vi "Test Get Skip Result.vi"(8 "error in (no error)":errorcluster, 11 "Test Case In":refnum<class "Test Case V2 Test.lvclass">) -> (0 "error out":errorcluster, 3 "Test Case Out":refnum<class "Test Case V2 Test.lvclass">)   [LabVIEW 2020, in "Test Case V2 Test.lvclass"]
uses:
  Test Case V2 Test.lvclass
  C:/Program Files (x86)/National Instruments/LabVIEW 2020/vi.lib/Astemes/LUnit/Test Case.lvclass
  LUnit Test Case V2 Test Double/LUnit Test Case V2 Test Double.lvclass
  C:/Git/astemes-lunit/source/Rewrite Project/LUnit Test Case/LUnit Test Case V2.lvclass
  Framework/Result Types/Assertion Result/Public/TypeDefs/Status.ctl
  <vilib>/Astemes/LUnit/Test Case.lvclass/Test Case.ctl
  d765b41f-6b96-4a08-8de0-d57f3ce312ff.vi
  <vilib>/Astemes/LUnit/Palette/Pass.vi
  <vilib>/Astemes/LUnit/Palette/Fail.vi
  <vilib>/Astemes/LUnit/Compare Variants.vi
  <vilib>/Astemes/LUnit/Describe Comparison.vi
  <vilib>/Astemes/LUnit/Set Assertion Type.vi
  <vilib>/Astemes/LUnit/Add test result.vi
  <vilib>/Astemes/LUnit/Variant to string.vi
  <vilib>/Astemes/LUnit/LUnit Record Assertion Result.vi
  <vilib>/Astemes/LUnit/LUnit Aggregate Assertion Results.vi
  <vilib>/Astemes/LUnit/Method Result/LUnit Merge Status.vi
  <vilib>/Astemes/LUnit/LUnit Concatenate result strings.vi
  <vilib>/Utility/Data Type/Get Type Information.vi
  <vilib>/Utility/LVClass/Get LV Class Name.vi
  LUnit Test Case/LUnit Test Case V2.lvclass
  Framework/Result Types/Assertion Result/Assertion Result.lvlib
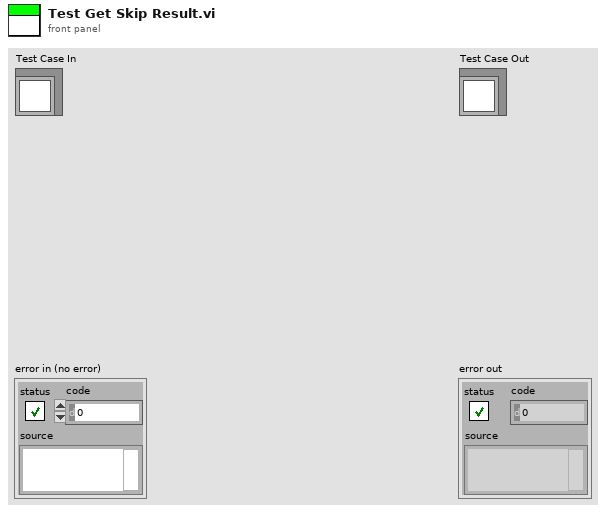
[diagram p1: front panel]
types:
  T1 = typedef "Assertion Result.lvlib/Status.ctl" = enum16{"Pass", "Fail", "Error", "Skipped", "Setup Error", "Broken", "Teardown Error"}
  T2 = typedef "Method Result.lvlib/Method Result.ctl" = cluster{"Test Case":string, "Test Method Name":string, "Status":T1, "Assertion Results":T3[], "Execution time":dbl, "Result String":string}
  T3 = typedef "Assertion Result.lvlib/Assertion Result.ctl" = cluster{"Status":T1, "Message":string, "Description":string, "Assertion Type":T4}
  T4 = typedef "Assertion Result.lvlib/Assertion Type.ctl" = enum16{"None", "Pass", "Fail", "Skip", "Pass if Equal", "Fail if Equal", "Pass if Error", "Fail if Error", "Pass if", "Fail if"}
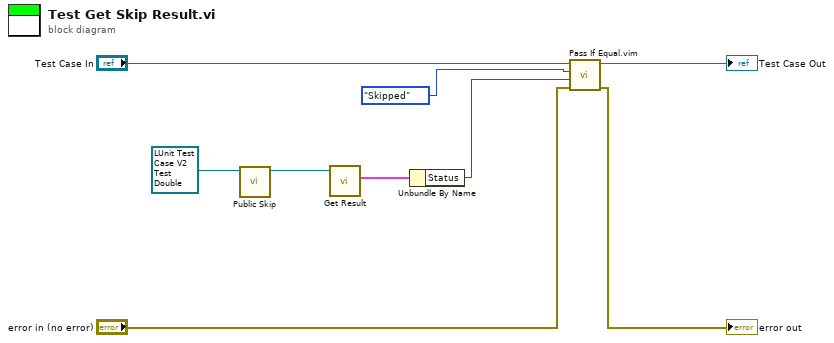
[diagram p0: block diagram]
diagram:
  n1 = call "Public Skip.vi"("LUnit Test Case V2 Test Double in"=refnum<class "LUnit Test Case V2 Test Double.lvclass"> refnum ("LUnit Test Case V2 Test Double.lvclass")) -> ("LUnit Test Case V2 Test Double out"=w4:refnum<class "LUnit Test Case V2 Test Double.lvclass">)  [unwired: 9 in, 1 out]
  n2 = call "Get Result.vi"("LUnit Test Case V2 In"=w4) -> ("Cluster of class private data"=w3:T2)  [unwired: 8 in, 2 out]
  n3 = Unbundle By Name(w3) -> ("Status"=w2:T1)
  n4 = call "Pass If Equal.vim"("error in (no error)"="error in (no error)", "Actual"=w2, "Expected"=Status."Skipped" ("Status"), "LUnit Test Case In"="Test Case In") -> ("error out"=→"error out":errorcluster, "LUnit Test Case Out"=→"Test Case Out":refnum<class "Test Case V2 Test.lvclass">)  [unwired: 6 in]
